vi "S706 parametrieren.vi"(8 "error in (no error)":errorcluster caption="Fehler (Eingang, kein Fehler)") -> (0 "error out":errorcluster caption="Fehler (Ausgang)")   [LabVIEW 2014]
uses:
  <vilib>/CANopenLib/CANOPEN.llb/CANopen SDO Create.vi
  <vilib>/CANopenLib/CANOPEN.llb/CANopen SDO Write [STR].vi
  <vilib>/CANopenLib/CANOPEN.llb/CANopen SDO Close.vi
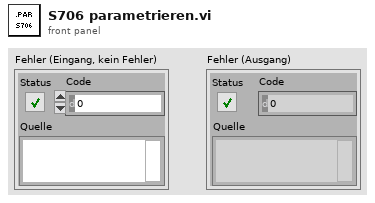
[diagram p1: front panel]
types:
  T1 = enum16{"unbekannt", "Quick stop active", "Fault reaction active", "Fault", "Operation enabled", "Switched on", "Ready to switch on", "Switch on disabled", "Not Ready to switch on"}
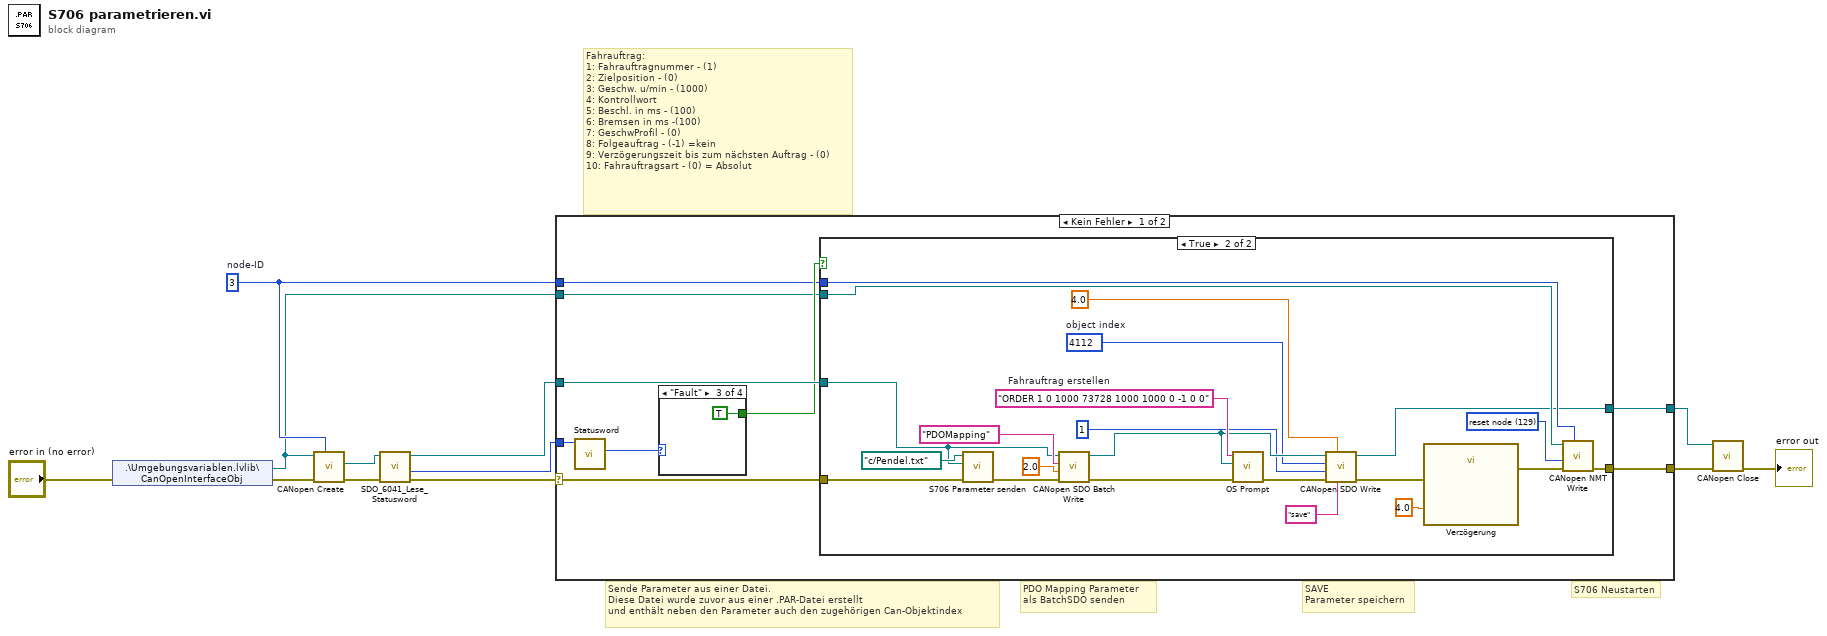
[diagram p0: block diagram]
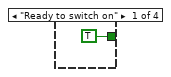
[diagram p3: hidden frame]
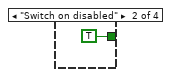
[diagram p4: hidden frame]
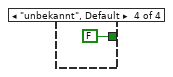
[diagram p5: hidden frame]
diagram:
  w2 = u8 3  # node-ID
  # "PDO Mapping Parameter\nals BatchSDO senden"
  # "Fahrauftrag:\n1: Fahrauftragnummer - (1)\n2: Zielposition - (0)\n3: Geschw. u/min - (1000)\n4: Kontrollwort\n5: Beschl. in ms - (100)\n6: Bremsen in ms -(100)\n7: GeschwProfil - (0)\n8: Folgeauftrag - (-1) =kein\n9: Verzögerungszeit bis zum nächsten Auftrag - (0)\n10: Fahrauftragsart - (0) = Absolut"
  # "S706 Neustarten"
  # "SAVE\nParameter speichern"
  # "Sende Parameter aus einer Datei.\nDiese Datei wurde zuvor aus einer .PAR-Datei erstellt\nund enthält neben den Parameter auch den zugehörigen Can-Objektindex"
  n1 = shared-variable ".\\Umgebungsvariablen.lvlib\\CanOpenInterfaceObj"(error in="error in (no error)") -> (w1:refnum<k20>, error out=w7:errorcluster)
  n2 = call-poly <vilib>:"CANopen Create.vi"("node-ID"=w2, "error in (no error)"=w7, "interface object in"=w1) -> ("error out"=w11:errorcluster, "SDO object out"=w12:refnum<k20>)  [unwired: 6 in, 1 out]
  n3 = call "SDO_6041_Lese_Statusword.vi"("error in (no error)"=w11, "SDO object in"=w12) -> ("error out"=w10:errorcluster, "U16 data"=w8:u16, "SDO object out"=w9:refnum<k20>)  [unwired: 6 in, 1 out]
  n4 = case shown="Kein Fehler" w10 {
    selector: w10 -> [w18 w51]
    tunnel: [w17 w51] -> w4
    tunnel: w9 -> [w19 w50]
    tunnel: w8 -> [w21 _]
    tunnel: [w13 w50] -> w3
    tunnel: w2 -> [w15 _]
    tunnel: w1 -> [w14 _]
    frame No Error {
      n5 = call "Statusword.vi"("Wert"=w21) -> ("Status"=w20:T1)  [unwired: 10 in]
      n6 = case shown="\"Fault\"" w20 {
        tunnel: [TRUE TRUE TRUE FALSE] -> w16
        frame "Ready to switch on" {
        }
        frame "Switch on disabled" {
        }
        frame "Fault" {
        }
        frame "unbekannt", Default {
        }
      }
      n7 = case shown="True" w16 {
        tunnel: w19 -> [w22 w33]
        tunnel: [w23 w38] -> w17
        tunnel: w18 -> [w23 w43]
        tunnel: w15 -> [_ w42]
        tunnel: w14 -> [_ w40]
        tunnel: [w22 w36] -> w13
        frame False {
        }
        frame True {
          w41 = u16 129 items=["start remote node"=1, "stop remote node"=2, "enter pre-operational"=128, "reset node"=129, "reset communication"=130] ("command")
          w26 = u16 4112  # object index
          w44 = "ORDER 1 0 1000 73728 1000 1000 0 -1 0 0"  # Fahrauftrag erstellen
          n8 = call "S706 Parameter senden.vi"("Fehler (Eingang)"=w43, "SDO object in"=w33, "Dateipfad (Dialog verwenden)"=path "c:/Pendel.txt") -> ("error out"=w35:errorcluster)  [unwired: 8 in]
          n9 = call <vilib>:"CANopen SDO Batch Write.vi"("error in (no error)"=w35, "timeout (1s)"=2.0, "batch SDO name"="PDOMapping", "SDO object in"=w33) -> ("error out"=w25:errorcluster, "SDO object out"=w28:refnum<k20>)  [unwired: 5 in, 1 out]
          n10 = call "OS Prompt.vi"("error"=w25, "SDO object in"=w28, "String"=w44) -> ("error out"=w34:errorcluster)  [unwired: 8 in]
          n11 = call-poly <vilib>:"CANopen SDO Write.vi"("string data"="save", "timeout (1s)"=4.0, "error in (no error)"=w34, "object sub-index (0)"=u8 1, "object index"=w26, "SDO object in"=w28) -> ("error out"=w31:errorcluster, "SDO object out"=w36:refnum<k20>)  [unwired: 3 in, 1 out]
          n12 = call "Verzögerung"("error in (no error)"=w31, "Delay Time (s)"=4.0) -> ("error out"=w30:errorcluster)  [unwired: 9 in]
          n13 = call <vilib>:"CANopen NMT Write.vi"("node-ID (0)"=w42, "error in (no error)"=w30, "command"=w41, "interface object in"=w40) -> ("error out"=w38:errorcluster)  [unwired: 6 in, 1 out]
        }
      }
    }
    frame Error {
    }
  }
  n14 = call-poly <vilib>:"CANopen Close.vi"("error in (no error)"=w4, "SDO object in"=w3) -> ("error out"=→"error out":errorcluster)  [unwired: 9 in]
